vi "GOOP_VirtualFolder_Item_Init.vi"(10 "Change Type":T1, 11 "Object":u64) -> ()   [LabVIEW 2014]
doc: "Copyright (c) 2010 Symbio (www.symbio.com). All rights reserved."
uses:
  <resource>/Framework/Providers/API/mxLvChangeType.ctl
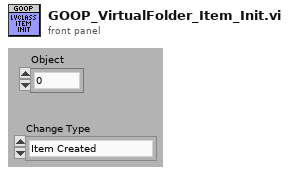
[diagram p1: front panel]
types:
  T1 = typedef "mxLvChangeType.ctl" = enum32{"Item Created", "Item Modified", "File Modified", "File Deleted", "Item Added", "Item Added to SCC", "Item Renamed", "Item Modified For SCC"}
  T2 = typedef "ItemRef.ctl" = u64
  T3 = typedef "AF_SettingsType.ctl" = cluster{"MessageFolderName":string}
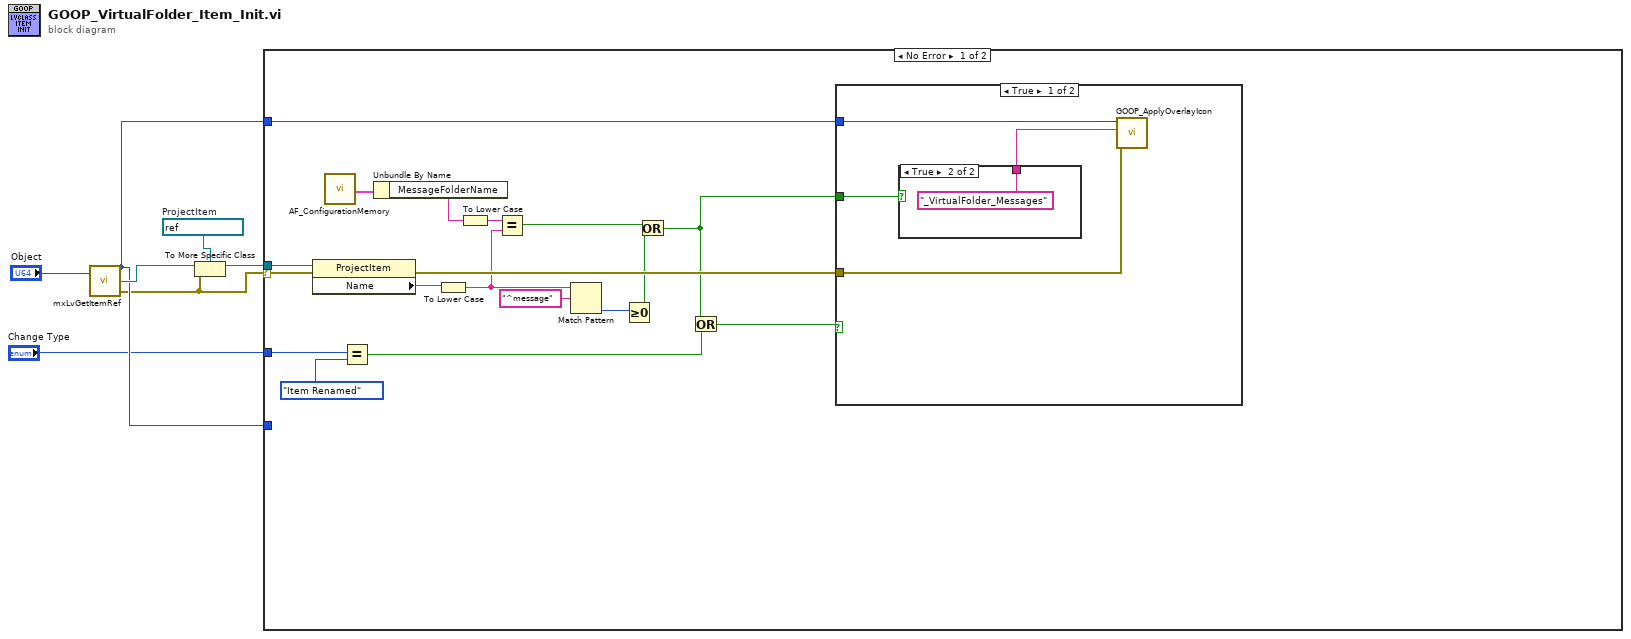
[diagram p0: block diagram]
diagram:
  w4 = refnum<vi> refnum  # ProjectItem
  n1 = call <resource>:"mxLvGetItemRef.vi"("Item"="Object") -> ("Item"=w3:T2, "Item Refnum"=w6:refnum<vi>, "error out"=w2:errorcluster)  [unwired: 1 in]
  n2 = To More Specific Class(target class=w4, reference=w6, error in=w2) -> (specific class reference=w5:refnum<vi>)  [unwired: 1 out]
  n3 = case shown="No Error" w2 {
    selector: w2 -> [w23 _]
    tunnel: w3 -> [w25 _]
    tunnel: w5 -> [w24 _]
    tunnel: w3 -> [_ _]
    tunnel: "Change Type" -> [w19 _]
    frame No Error {
      n4 = property class="ProjectItem"(reference=w24, error in=w23) -> (error out=w22:errorcluster, "Name"=w20:string)  [unwired: 1 out]
      n5 = call <resource>:"AF_ConfigurationMemory.vi"() -> ("AF_SettingsOut"=w14:T3)  [unwired: 16 in, 3 out]
      n6 = Equal?(x=w19, y=mxLvChangeType."Item Renamed") -> (x = y?=w16:bool)
      n7 = Unbundle By Name(w14) -> ("MessageFolderName"=w13:string)
      n8 = To Lower Case(string=w20) -> (all lower case string=w11:string)
      n9 = To Lower Case(string=w13) -> (all lower case string=w12:string)
      n10 = Equal?(x=w12, y=w11) -> (x = y?=w10:bool)
      n11 = Match Pattern(string=w11, regular expression="^message") -> (offset past match=w17:i32)  [unwired: 1 in, 3 out]
      n12 = Greater Or Equal To 0?(x=w17) -> (x >= 0?=w9:bool)
      n13 = Or(x=w10, y=w9) -> (x .or. y?=w8:bool)
      n14 = Or(x=w8, y=w16) -> (x .or. y?=w15:bool)
      n15 = case shown="True" w15 {
        tunnel: w25 -> [w29 _]
        tunnel: w22 -> [w27 _]
        tunnel: w8 -> [w26 _]
        frame True {
          n16 = case shown="True" w26 {
            tunnel: [_ "_VirtualFolder_Messages" ("ClassItemIconName(NoExtension)")] -> w28
            frame False {
            }
            frame True {
            }
          }
          n17 = call <resource>:"GOOP_ApplyOverlayIcon.vi"("error in (no error)"=w27, "IconName(NoPngExtension)"=w28, "Object"=w29) -> ()  [unwired: 8 in, 1 out]
        }
        frame False {
        }
      }
    }
    frame Error {
    }
  }
